vi "실습 2-9 absolute Position.vi"() -> ()   [LabVIEW 2014]
uses:
  <vilib>/Motion/FlexMotion/CustomControls/CustomControls.llb/AxisOrVectorSpace To Configure.flx
  <vilib>/Motion/FlexMotion/FunctionsVIs/StartStopMotion.llb/Start Motion (8 axes).flx
  <vilib>/Motion/FlexMotion/FunctionsVIs/StartStopMotion.llb/Stop Motion (8 axes).flx
panel:
  in  "정지":bool
  out "Position":i32
  in  "Target Position (0)":i32=-36000
  in  "Velocity (10000)":i32=3600
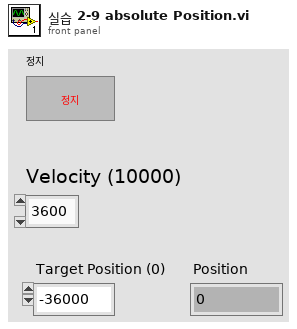
[diagram p1: front panel]
types:
  T1 = enum16{"Absolute Position", "Relative Position", "Velocity", "Relative to Cap Pos", "Modulus Position", "Absolute Contouring", "Relative Contouring"}
  T2 = typedef "AxisOrVectorSpace To Configure.flx" = u16
  T3 = typedef "Resource Out (Enum).flx" = u16
  T4 = typedef "Bd Id Out" = u8
  T5 = cluster{"Run/Stop":bool, "Profile Complete":bool, "Motor Off ":bool, "Following Error":bool, "Limit Switch":bool, "Home Switch":bool, "SW Limit Switch":bool, "Watchdog":bool, "Velocity Threshold":bool, "Position Brkpt":bool, "Home Found":bool, "Index Found":bool, "High Speed Capture":bool, "Reverse Direction":bool, "Blend Complete":bool, "Move Complete":bool}
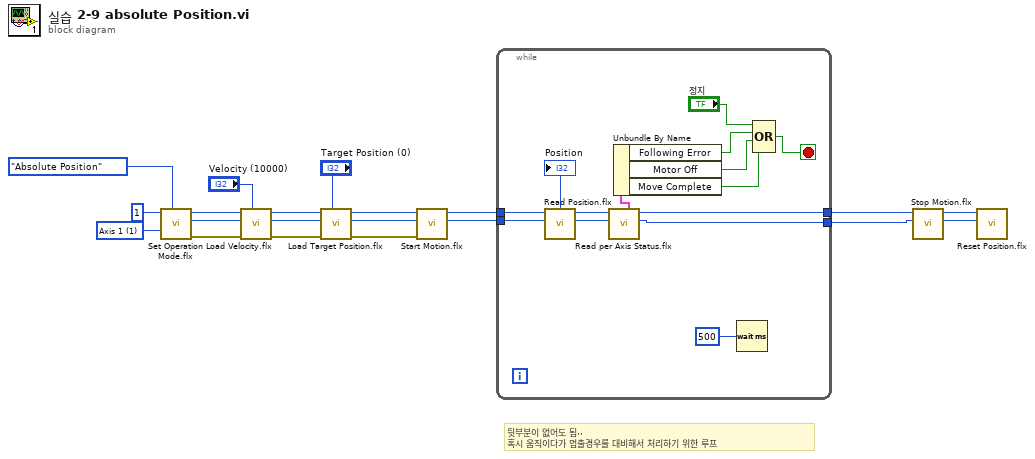
[diagram p0: block diagram]
diagram:
  w19 = T2 1 items=["Axis 1"=1, "Axis 2"=2, "Axis 3"=3, "Axis 4"=4, "Axis 5"=5, "Axis 6"=6, "Axis 7"=7, "Axis 8"=8, "Vector Space 1"=17, "Vector Space 2"=18, "Vector Space 3"=19, "Vector Space 4"=20] ("Axis or Vector Space")
  # "뒷부분이 없어도 됨,,\n혹시 움직이다가 멈출경우를 대비해서 처리하기 위한 루프"
  n1 = call <vilib>:"Set Operation Mode.flx"("Position Mode (Absolute)"=T1."Absolute Position", "Axis or Vector Space"=w19, "Board ID"=u8 1) -> ("error out"=w14:errorcluster, "Resource Output"=w15:T3, "Bd ID Out"=w16:T4)  [unwired: 3 in]
  n2 = call <vilib>:"Load Velocity.flx"("Velocity (10000)"="Velocity (10000)", "error in (no error)"=w14, "Axis or Vector Space"=w15, "Board ID"=w16) -> ("error out"=w11:errorcluster, "Resource Output"=w12:T3, "Bd ID Out"=w13:T4)  [unwired: 3 in]
  n3 = call <vilib>:"Load Target Position.flx"("Target Position (0)"="Target Position (0)", "error in (no error)"=w11, "Axis"=w12, "Board ID"=w13) -> ("error out"=w8:errorcluster, "Resource Output"=w9:T3, "Bd ID Out"=w10:T4)  [unwired: 3 in]
  n4 = call-poly <vilib>:"Start Motion.flx"("error in (no error)"=w8, "Axis or Vector Space"=w9, "Board ID"=w10) -> ("Resource Output"=w5:T3, "Bd ID Out"=w6:T4)  [unwired: 3 in, 1 out]
  n5 = while {
    tunnel: w6 -> [w34]
    tunnel: w5 -> [w33]
    tunnel: [w29] -> w4
    tunnel: [w28] -> w3
    stop <- w22 stop-if-true
    n6 = call <vilib>:"Read Position.flx"("Axis"=w33, "Board ID"=w34) -> ("Resource Output"=w31:T3, "Bd ID Out"=w32:T4, "Position"=→"Position":i32)  [unwired: 4 in, 1 out]
    n7 = call <vilib>:"Read per Axis Status.flx"("Axis"=w31, "Board ID"=w32) -> ("Resource Output"=w28:T3, "Bd ID Out"=w29:T4, "Per Axis H/W Status"=w30:T5)  [unwired: 4 in, 1 out]
    n8 = Unbundle By Name(w30) -> ("Following Error"=w27:bool, "Motor Off"=w26:bool, "Move Complete"=w25:bool)
    n9 = Wait (ms)(milliseconds to wait=u32 500 ("대기 시간(ms)")) -> ()  [unwired: 1 out]
    n10 = Compound Arithmetic op=OR("정지", w27, w26, w25) -> (w22:bool)
  }
  n11 = call-poly <vilib>:"Stop Motion.flx"("Axis or Vector Space"=w3, "Board ID"=w4) -> ("Resource Output"=w1:T3, "Bd ID Out"=w2:T4)  [unwired: 5 in, 1 out]
  n12 = call <vilib>:"Reset Position.flx"("Axis"=w1, "Board ID"=w2) -> ()  [unwired: 5 in, 3 out]
